vi "FPGA_AnalogTriggerWriteUpperLimit.vi"(8 "error in (no error)":errorcluster, 10 "UpperLimit":i32, 11 "AnalogTriggerDevRef":T1) -> (0 "error out":errorcluster, 3 "AnalogTriggerDevRef":T1)   [LabVIEW 2017]
uses:
  <vilib>/Rock Robotics/SystemInterfaces/AnalogTrigger/FPGA_AnalogTriggerDevRef.ctl
  <vilib>/Rock Robotics/SystemInterfaces/AnalogTrigger/FPGA_AnalogTriggerIndex.ctl
  <vilib>/rvi/errors/niLvFpgaAdjustHostInterfaceError.vi
  <vilib>/Utility/error.llb/Error Cluster From Error Code.vi
  <vilib>/Rock Robotics/SystemInterfaces/System/FPGA_SystemFPGA Ref Global.vi
  <vilib>/Rock Robotics/SystemInterfaces/System/FPGA_SystemFRC FPGA Ref.ctl
  <vilib>/rvi/interface/nirviReadWriteControl/nirviReadWriteControl.xnode
  NiFpgaLv.dll
  <vilib>/rvi/interface/Simulation/niFpgaSimulationCallBeginRW.vi
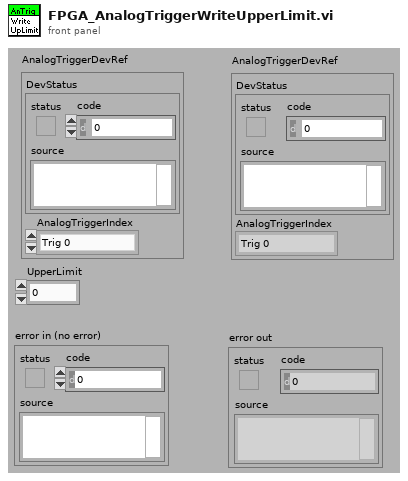
[diagram p1: front panel]
types:
  T1 = typedef "FPGA_AnalogTriggerDevRef.ctl" = cluster{"DevStatus":errorcluster, "AnalogTriggerIndex":T2}
  T2 = typedef "FPGA_AnalogTriggerIndex.ctl" = enum8{"Trig 0", "Trig 1", "Trig 2", "Trig 3", "Trig 4", "Trig 5", "Trig 6", "Trig 7", "Invalid"}
  T3 = typedef "FPGA_SystemFRC FPGA Ref.ctl" = refnum<k20>
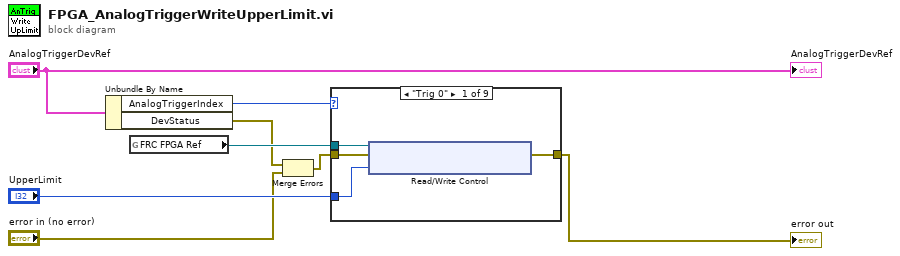
[diagram p0: block diagram]
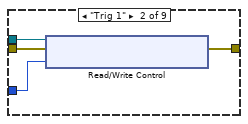
[diagram p2: hidden frame]
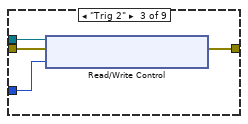
[diagram p3: hidden frame]
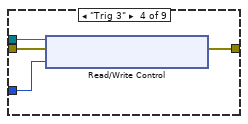
[diagram p4: hidden frame]
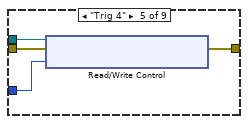
[diagram p5: hidden frame]
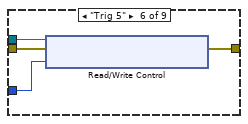
[diagram p6: hidden frame]
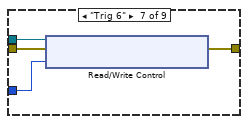
[diagram p7: hidden frame]
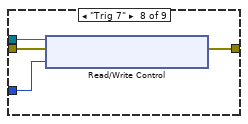
[diagram p8: hidden frame]
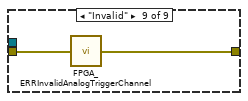
[diagram p9: hidden frame]
diagram:
  n1 = Unbundle By Name("AnalogTriggerDevRef") -> ("AnalogTriggerIndex"=w5:T2, "DevStatus"=w3:errorcluster)
  n2 = global read "FPGA_SystemFPGA Ref Global.vi" "FRC FPGA Ref"() -> (w4:T3)
  n3 = Merge Errors(w3, "error in (no error)") -> (w2:errorcluster)
  n4 = case shown="\"Trig 0\"" w5 {
    tunnel: w4 -> [w11 w16 w20 w24 w28 w32 w36 w40 _]
    tunnel: w2 -> [w12 w15 w19 w23 w27 w31 w35 w39 w42]
    tunnel: [w10 w14 w18 w22 w26 w30 w34 w38 w41] -> w8
    tunnel: "UpperLimit" -> [w9 w13 w17 w21 w25 w29 w33 w37 _]
    frame "Trig 0" {
      n5 = xnode "Read/Write Control"("FPGA VI Reference In"=w11, "error in"=w12, "AnalogTrigger0.UpperLimit"=w9) -> ("error out"=w10:errorcluster)  [unwired: 1 out]
    }
    frame "Trig 1" {
      n6 = xnode "Read/Write Control"("FPGA VI Reference In"=w16, "error in"=w15, "AnalogTrigger1.UpperLimit"=w13) -> ("error out"=w14:errorcluster)  [unwired: 1 out]
    }
    frame "Trig 2" {
      n7 = xnode "Read/Write Control"("FPGA VI Reference In"=w20, "error in"=w19, "AnalogTrigger2.UpperLimit"=w17) -> ("error out"=w18:errorcluster)  [unwired: 1 out]
    }
    frame "Trig 3" {
      n8 = xnode "Read/Write Control"("FPGA VI Reference In"=w24, "error in"=w23, "AnalogTrigger3.UpperLimit"=w21) -> ("error out"=w22:errorcluster)  [unwired: 1 out]
    }
    frame "Trig 4" {
      n9 = xnode "Read/Write Control"("FPGA VI Reference In"=w28, "error in"=w27, "AnalogTrigger4.UpperLimit"=w25) -> ("error out"=w26:errorcluster)  [unwired: 1 out]
    }
    frame "Trig 5" {
      n10 = xnode "Read/Write Control"("FPGA VI Reference In"=w32, "error in"=w31, "AnalogTrigger5.UpperLimit"=w29) -> ("error out"=w30:errorcluster)  [unwired: 1 out]
    }
    frame "Trig 6" {
      n11 = xnode "Read/Write Control"("FPGA VI Reference In"=w36, "error in"=w35, "AnalogTrigger6.UpperLimit"=w33) -> ("error out"=w34:errorcluster)  [unwired: 1 out]
    }
    frame "Trig 7" {
      n12 = xnode "Read/Write Control"("FPGA VI Reference In"=w40, "error in"=w39, "AnalogTrigger7.UpperLimit"=w37) -> ("error out"=w38:errorcluster)  [unwired: 1 out]
    }
    frame "Invalid" {
      n13 = call <vilib>:"FPGA_ERRInvalidAnalogTriggerChannel.vi"("error in (no error)"=w42) -> ("error out"=w41:errorcluster)
    }
  }
  "error out" <- w8
  "AnalogTriggerDevRef" <- "AnalogTriggerDevRef"
